vi "ReadPortsHeader.vi"(0 "base path":path, 1 "FileName":string) -> (2 "Output Names":string[](array[string]), 3 "Input Names":string[](array[string]), 4 "Output Numbers":i32[](array[numeric]), 5 "Input Numbers":i32[](array[numeric]))   [LabVIEW 2019]
panel:
  out "before substring":string
  out "after substring":string
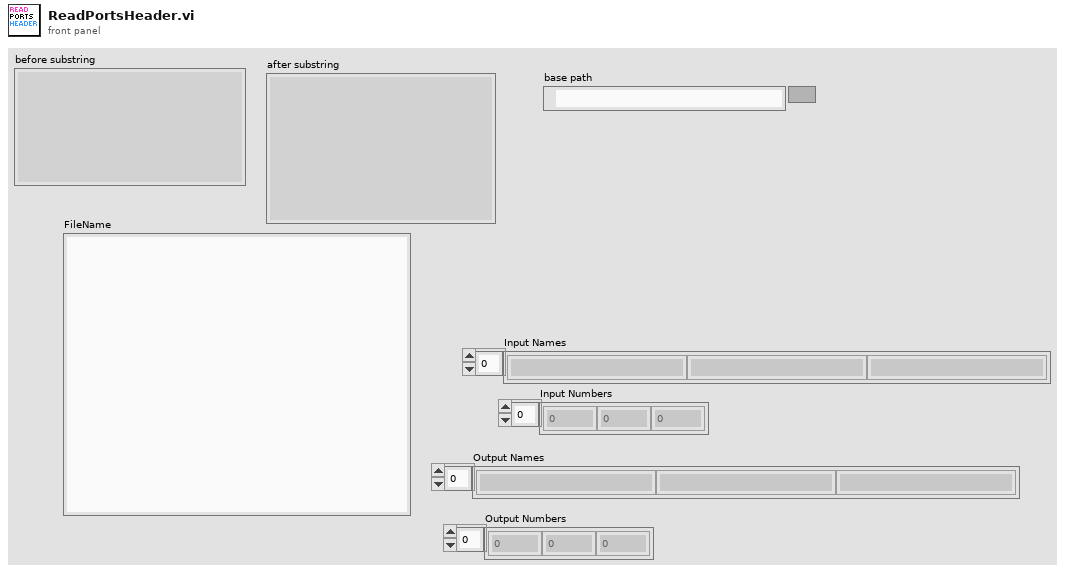
[diagram p1: front panel]
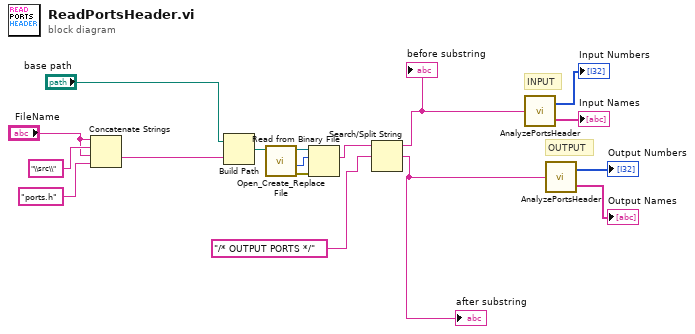
[diagram p0: block diagram]
diagram:
  # "OUTPUT"
  # "INPUT"
  n1 = Concatenate Strings("FileName", "\\src\\" ("string"), "FileName", "ports.h" ("name or relative path")) -> (w5:string)
  n2 = Build Path(base path="base path", name or relative path=w5) -> (appended path=w10:path)
  n3 = call <vilib>:"Open_Create_Replace File.vi"("file path"=w10) -> ("error out"=w11:errorcluster, "file size (bytes)"=w12:i32, "refnum"=w13:refnum<file>)  [unwired: 7 in, 1 out]
  n4 = Read from Binary File(8:w11, 10:w12, 11:w13) -> (2:w4:string)  [unwired: 3 in, 3 out]
  n5 = Search/Split String(string=w4, search string/char (-)="/* OUTPUT PORTS */" ("regular expression")) -> (substring before match=w2:string, match + rest of string=w1:string)  [unwired: 1 in, 1 out]
  "after substring" <- w1
  "before substring" <- w2
  n6 = call "AnalyzePortsHeader.vi"("data"=w2) -> ("Input Names"=→"Input Names":string[], "Input Numbers"=→"Input Numbers":i32[])
  n7 = call "AnalyzePortsHeader.vi"("data"=w1) -> ("Input Names"=→"Output Names":string[], "Input Numbers"=→"Output Numbers":i32[])
